vi "Read threshold.vi"(8 "error in (no error)":errorcluster, 11 "SetGlobalThreshold in":refnum<class "SetGlobalThresholdMsg.lvclass">) -> (0 "error out":errorcluster, 2 "Severity":T1=enum."INFO", 3 "SetGlobalThreshold out":refnum<class "SetGlobalThresholdMsg.lvclass">)   [LabVIEW 2026, in "Lumberjack.lvlib" / "SetGlobalThresholdMsg.lvclass"]
doc: "Returns the Severity threshold carried by this SetGlobalThresholdMsg.\nClass private-data accessor; reads the message's `threshold` field with no side effects.\nLumberjack.lvlib, SetGlobalThresholdMsg.lvclass, public."
uses:
  SetGlobalThresholdMsg.lvclass
  TypeDefs/Severity.ctl
  SetGlobalThresholdMsg.lvclass/SetGlobalThresholdMsg.ctl
  Lumberjack.lvlib
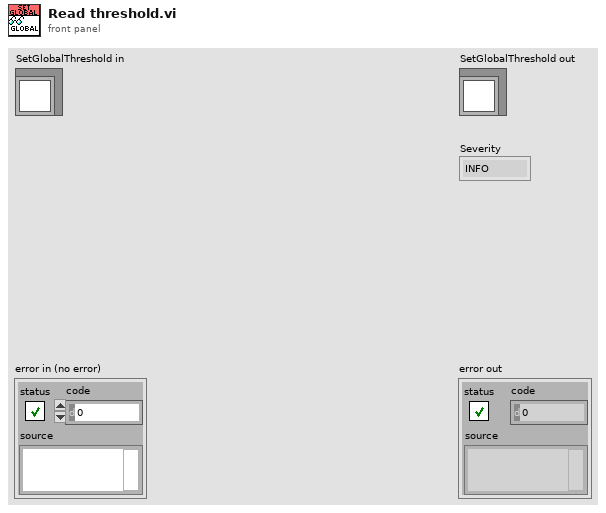
[diagram p1: front panel]
types:
  T1 = typedef "Lumberjack.lvlib/Severity.ctl" = enum16{"OFF", "FATAL", "ERROR", "WARN", "INFO", "DEBUG", "TRACE", "ALL"}
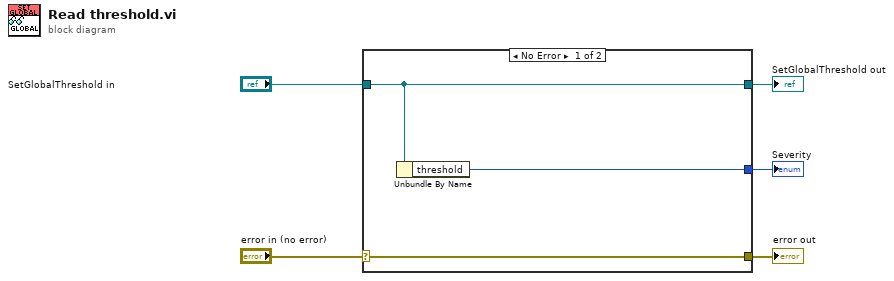
[diagram p0: block diagram]
diagram:
  n1 = case shown="No Error" "error in (no error)" {
    selector: "error in (no error)" -> [w8 w9]
    tunnel: [w8 w9] -> w4
    tunnel: [w7 w10] -> w2
    tunnel: "SetGlobalThreshold in" -> [w7 w10]
    tunnel: [w6 _] -> w1
    frame No Error {
      n2 = Unbundle By Name(w7) -> ("threshold"=w6:T1)
    }
    frame Error {
    }
  }
  "error out" <- w4
  "SetGlobalThreshold out" <- w2
  "Severity" <- w1
